vi "啮合.vi"(8 "error in (no error)":errorcluster caption="错误输入（无错误）", 11 "信号数据":dbl[][](array[numeric])) -> (0 "error out":errorcluster caption="错误输出")   [LabVIEW 2015, in "Logging.lvlib"]
uses:
  Logging.lvlib
panel:
  out "反转扭矩变化峰值":dbl
  out "反转最小值":dbl
  out "反转最大值":dbl
  out "扭矩反转平均值":dbl
  out "左右变化值":dbl
  out "正转扭矩变化峰值":dbl
  out "正转最小值":dbl
  out "正转最大值":dbl
  out "扭矩正转平均值":dbl
  out "总圈数":dbl
  in  "取消按钮":bool
  in  "确定按钮":bool
  # "啮合测量结果"
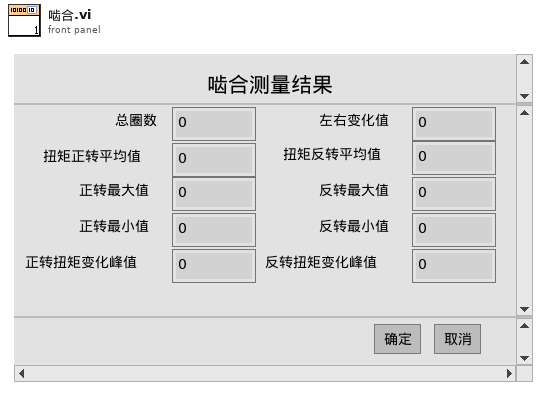
[diagram p1: front panel]
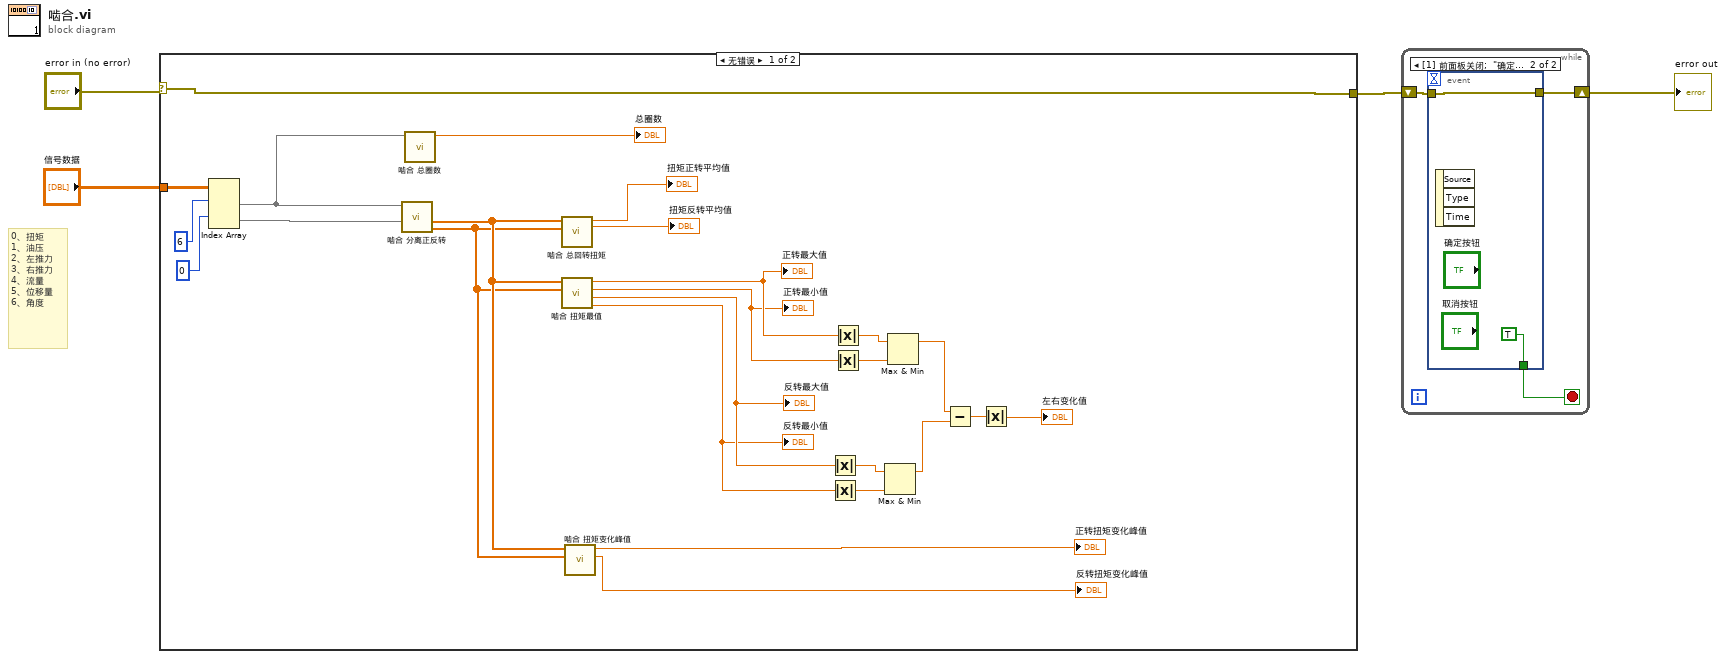
[diagram p0: block diagram]
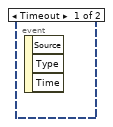
[diagram p2: hidden frame]
diagram:
  # "0、扭矩\n1、油压\n2、左推力\n3、右推力\n4、流量\n5、位移量\n6、角度"
  n1 = case shown="无错误" "error in (no error)" {
    selector: "error in (no error)" -> [w7 w30]
    tunnel: "信号数据" -> [w29 _]
    tunnel: [w7 w30] -> w1
    frame No Error {
      n2 = Index Array(array=w29, index (row) #1=6 ("禁用的索引 (列)"), index (row) #2=0 ("索引 (行)")) -> (element #1=w25:dbl[], element #2=w26:dbl[])  [unwired: 2 in]
      n3 = call "啮合 分离正反转.vi"("输入扭矩"=w26, "输入角度"=w25) -> ("扭矩反转"=w5:dbl[], "扭矩正转"=w6:dbl[])  [unwired: 6 in, 2 out]
      n4 = call "啮合 总圈数.vi"("输入角度"=w25) -> ("总圈数"=→"总圈数":dbl)  [unwired: 10 in]
      n5 = call "啮合 总回转扭矩.vi"("扭矩反转"=w5, "扭矩正转"=w6) -> ("扭矩反转平均值"=→"扭矩反转平均值":dbl, "扭矩正转平均值"=→"扭矩正转平均值":dbl)  [unwired: 8 in]
      n6 = call "啮合 扭矩最值.vi"("扭矩正转"=w5, "扭矩反转"=w6) -> ("反转最小值"=w14:dbl, "反转最大值"=w15:dbl, "正转最小值"=w20:dbl, "正转最大值"=w21:dbl)  [unwired: 6 in]
      "正转最大值" <- w21
      "正转最小值" <- w20
      "反转最大值" <- w15
      "反转最小值" <- w14
      n7 = call "啮合 扭矩变化峰值.vi"("扭矩反转"=w5, "扭矩正转"=w6) -> ("反转扭矩变化峰值"=→"反转扭矩变化峰值":dbl, "正转扭矩变化峰值"=→"正转扭矩变化峰值":dbl)  [unwired: 8 in]
      n8 = Absolute Value(x=w15) -> (abs(x)=w16:dbl)
      n9 = Absolute Value(x=w14) -> (abs(x)=w17:dbl)
      n10 = Absolute Value(x=w21) -> (abs(x)=w18:dbl)
      n11 = Absolute Value(x=w20) -> (abs(x)=w19:dbl)
      n12 = Max & Min(x=w16, y=w17) -> (max(x,y)=w12:dbl)  [unwired: 1 out]
      n13 = Max & Min(x=w18, y=w19) -> (max(x,y)=w13:dbl)  [unwired: 1 out]
      n14 = Subtract(x=w13, y=w12) -> (x-y=w11:dbl)
      n15 = Absolute Value(x=w11) -> (abs(x)=→"左右变化值":dbl)
    }
    frame Error {
    }
  }
  n16 = while {
    shift-right: [w33] -> w2
    shift-left: w1 -> [w32]
    stop <- w31 stop-if-true
    n17 = event shown="[1] 前面板关闭;  \"确定按钮\", \"取消按钮\": 值改变" {
      selector: _ -> [_ _]
      dyn-events: _ -> [_ _]
      timeout: _ -> [_ _]
      tunnel: [_ w35] -> w33
      tunnel: w32 -> [_ w35]
      tunnel: [_ TRUE] -> w31
      event Timeout {
        n18 = event-data() -> ()  [unwired: 1 in, 3 out]
      }
      event Panel Close; "确定按钮", "取消按钮": Value Change {
        n19 = event-data() -> ()  [unwired: 1 in, 3 out]
      }
    }
  }
  "error out" <- w2
